vi "FormatPositions.vi"(1 "Pos Info":T1) -> (0 "Pos strings":string[](array[string]))   [LabVIEW 2015]
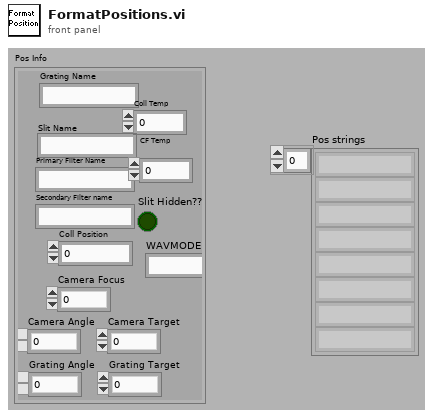
[diagram p1: front panel]
types:
  T1 = cluster{"Grating Name":string, "Slit Name":string, "Primary Filter Name":string, "Secondary Filter name":string, "Coll Position":i32, "Camera Focus":i32, "Camera Angle":dbl, "Grating Angle":dbl, "Coll Temp":dbl, "CF Temp\n":dbl, "Camera Target":dbl, "Grating Target":dbl, "WAVMODE":string, "Slit Hidden??":bool}
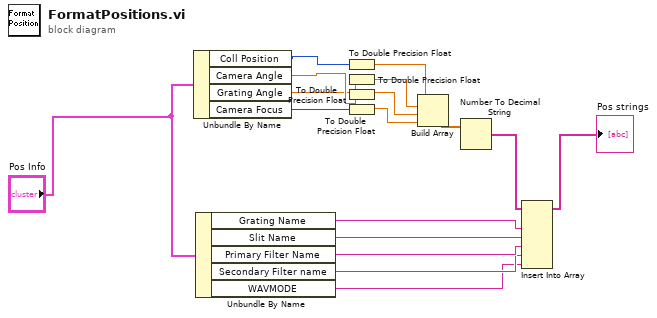
[diagram p0: block diagram]
diagram:
  n1 = Unbundle By Name("Pos Info") -> ("Coll Position"=w12:i32, "Camera Angle"=w11:dbl, "Grating Angle"=w10:dbl, "Camera Focus"=w9:i32)
  n2 = Unbundle By Name("Pos Info") -> ("Grating Name"=w6:string, "Slit Name"=w5:string, "Primary Filter Name"=w4:string, "Secondary Filter name"=w3:string, "WAVMODE"=w2:string)
  n3 = To Double Precision Float(number=w12) -> (double precision float=w17:dbl)
  n4 = To Double Precision Float(number=w11) -> (double precision float=w16:dbl)
  n5 = To Double Precision Float(number=w10) -> (double precision float=w15:dbl)
  n6 = To Double Precision Float(number=w9) -> (double precision float=w14:dbl)
  n7 = Build Array(w17, w16, w15, w14) -> (w13:dbl[])
  n8 = Number To Decimal String(number=w13) -> (decimal integer string=w7:string[])  [unwired: 1 in]
  n9 = Insert Into Array(array=w7, new element #1=w6, new element #2=w5, new element #3=w4, new element #4=w3, new element #5=w2) -> (→"Pos strings":string[])  [unwired: 1 in]
